vi "ADAM_to_Eng_units.vi"(3 "Ch Description":T1={"Ch Name"="", "Type"="", "Function"=enum."Analogue Input", "Ch State"=enum."On", "Calibration type"="", "A"=0.0, "B"=0.0, "C"=0.0, "D"=0.0, "Comments"="", "Address"={"Main"=0, "Ch."=0, "Sub"=0, "Port Name"=""}, "String"="", "Duty"=65535} {"Duty" format="%016b"; "D" format="%#_5g"; "C" format="%#_5g"; "B" format="%#_5g"; "A" format="%#_5g"}, 5 "Raw":dbl format="%.2f") -> (1 "Calibrated units":dbl format="%.2f", 2 "Comments":string)   [LabVIEW 2021]
uses:
  ADAM Client/Sub VIs/ADAM Controls/Ch_description_ADAM.ctl
  ADAM Client/Sub VIs/ADAM Controls/Module_type_ADAM.ctl
  ADAM Client/Sub VIs/ADAM Controls/Function_ADAM.ctl
  ADAM Client/Sub VIs/ADAM Controls/Channel_State.ctl
  ADAM Client/Sub VIs/ADAM Controls/Calib_type_ADAM.ctl
  ADAM Client/Sub VIs/ADAM Controls/Address.ctl
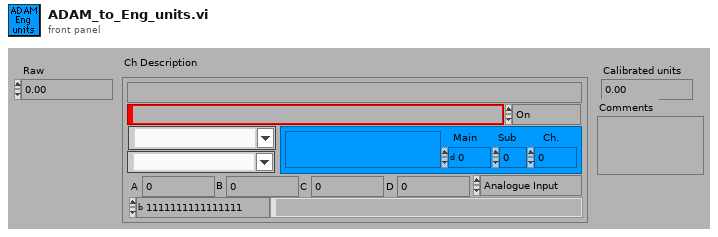
[diagram p1: front panel]
types:
  T1 = typedef "Ch_description_ADAM.ctl" = cluster{"Ch Name":string, "Type":T2, "Function":T3, "Ch State":T4, "Calibration type":T5, "A":dbl, "B":dbl, "C":dbl, "D":dbl, "Comments":string, "Address":T6, "String":string, "Duty":u16}
  T2 = typedef "Module_type_ADAM.ctl" = string
  T3 = typedef "Function_ADAM.ctl" = enum16{"Analogue Input", "Digital Input", "Event counter", "Event rate", "Analogue Output", "Digital Output", "Relay Output"}
  T4 = typedef "Channel_State.ctl" = enum16{"On", "Off", "Always On", "Always Off"}
  T5 = typedef "Calib_type_ADAM.ctl" = string
  T6 = typedef "Address.ctl" = cluster{"Main":i32, "Ch.":i32, "Sub":i32, "Port Name":string}
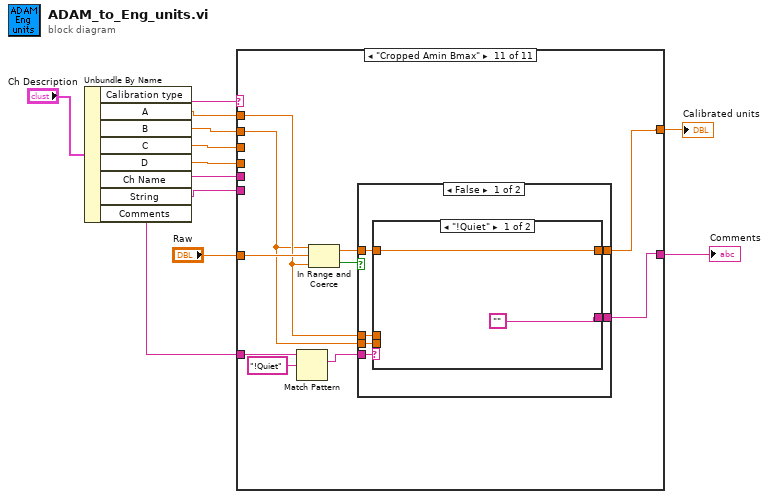
[diagram p0: block diagram]
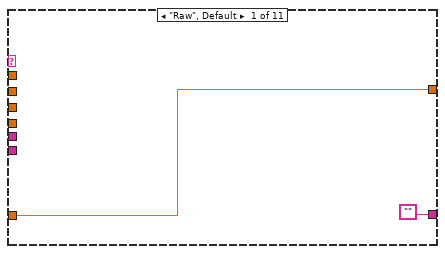
[diagram p2: hidden frame]
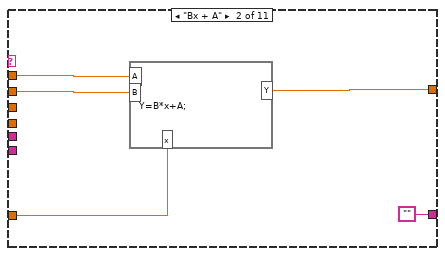
[diagram p3: hidden frame]
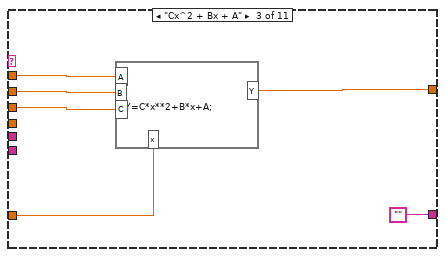
[diagram p4: hidden frame]
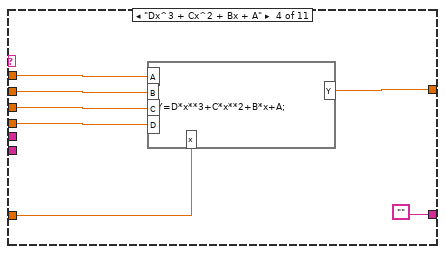
[diagram p5: hidden frame]
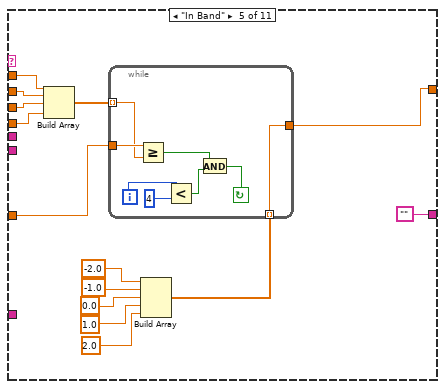
[diagram p6: hidden frame]
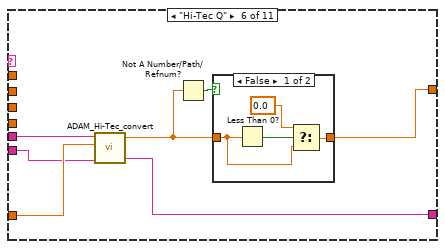
[diagram p7: hidden frame]
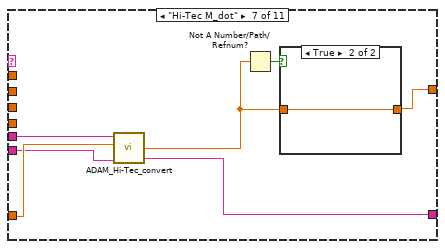
[diagram p9: hidden frame]
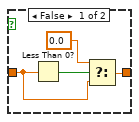
[diagram p10: hidden frame]
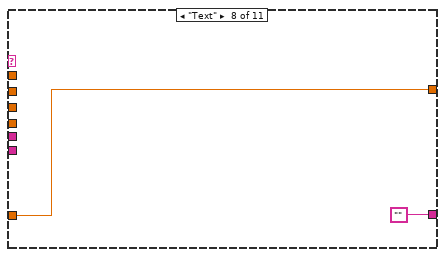
[diagram p11: hidden frame]
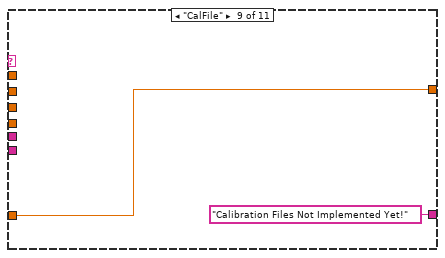
[diagram p12: hidden frame]
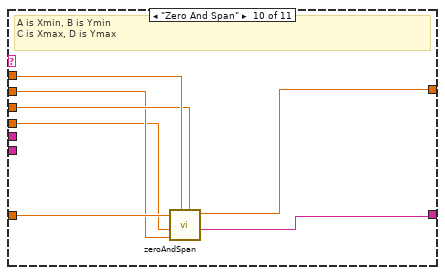
[diagram p13: hidden frame]
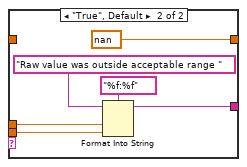
[diagram p14: hidden frame]
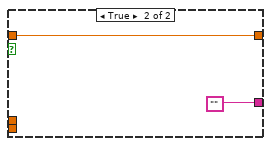
[diagram p15: hidden frame]
diagram:
  n1 = Unbundle By Name("Ch Description") -> ("Calibration type"=w11:T5, "A"=w8:dbl, "B"=w7:dbl, "C"=w6:dbl, "D"=w5:dbl, "Ch Name"=w4:string, "String"=w2:string, "Comments"=w1:string)
  n2 = case shown="\"Cropped Amin Bmax\"" w11 {
    tunnel: [w14 w19 w25 w32 w35 w58 w70 w80 w82 w87 w97] -> w10
    tunnel: "Raw" -> [w14 w16 w21 w27 w42 w60 w72 w80 w82 w89 w99]
    tunnel: w8 -> [_ w18 w24 w31 w46 _ _ _ _ w86 w94]
    tunnel: w7 -> [_ w17 w23 w30 w45 _ _ _ _ w84 w93]
    tunnel: w6 -> [_ _ w22 w29 w44 _ _ _ _ w85 _]
    tunnel: w5 -> [_ _ _ w28 w43 _ _ _ _ w83 _]
    tunnel: w4 -> [_ _ _ _ _ w61 w73 _ _ _ _]
    tunnel: ["" "" "" "" "" w56 w68 "" "Calibration Files Not Implemented Yet!" ("Comments") w88 w95] -> w3
    tunnel: w2 -> [_ _ _ _ _ w55 w67 _ _ _ _]
    tunnel: w1 -> [_ _ _ _ _ _ _ _ _ _ w91]
    frame "Raw", Default {
    }
    frame "Bx + A" {
      n3 = formula code="Y=B*x+A;"("A"=w18, "B"=w17, "x"=w16) -> ("Y"=w19:dbl)
    }
    frame "Cx^2 + Bx + A" {
      n4 = formula code="Y=C*x**2+B*x+A;"("A"=w24, "B"=w23, "C"=w22, "x"=w21) -> ("Y"=w25:dbl)
    }
    frame "Dx^3 + Cx^2 + Bx + A" {
      n5 = formula code="Y=D*x**3+C*x**2+B*x+A;"("A"=w31, "B"=w30, "C"=w29, "D"=w28, "x"=w27) -> ("Y"=w32:dbl)
    }
    frame "In Band" {
      n6 = Build Array(w46, w45, w44, w43) -> (w41:dbl[])
      n7 = Build Array(-2.0, -1.0, 0.0, 1.0, 2.0) -> (w34:dbl[])
      n8 = while {
        tunnel: w34 -> [w52] mode=indexing
        tunnel: [w52] -> w35
        tunnel: w41 -> [w53] mode=indexing
        tunnel: w42 -> [w54]
        i -> [w51]
        stop <- w47 continue-if-true
        n9 = Greater Or Equal?(x=w54, y=w53) -> (x >= y?=w48:bool)
        n10 = Less?(x=w51, y=4) -> (x < y?=w49:bool)
        n11 = And(x=w48, y=w49) -> (x .and. y?=w47:bool)
      }
    }
    frame "Hi-Tec Q" {
      n12 = call "ADAM_Hi-Tec_convert.vi"("Ch Name"=w61, "Raw"=w60, "Channel Read"=w55) -> ("Q release (l/min)"=w57:dbl, "Comments"=w56:string)  [unwired: 1 in, 2 out]
      n13 = Not A Number/Path/Refnum?(number/path/refnum=w57) -> (NaN/Path/Refnum?=w59:bool)
      n14 = case shown="False" w59 {
        tunnel: [w63 w66] -> w58
        tunnel: w57 -> [w64 w66]
        frame False {
          n15 = Less Than 0?(x=w64) -> (x < 0?=w65:bool)
          n16 = Select(t=0.0, s=w65, f=w64) -> (s? t:f=w63:dbl)
        }
        frame True {
        }
      }
    }
    frame "Hi-Tec M_dot" {
      n17 = call "ADAM_Hi-Tec_convert.vi"("Ch Name"=w73, "Raw"=w72, "Channel Read"=w67) -> ("M_dot (kg/min)"=w69:dbl, "Comments"=w68:string)  [unwired: 1 in, 2 out]
      n18 = Not A Number/Path/Refnum?(number/path/refnum=w69) -> (NaN/Path/Refnum?=w71:bool)
      n19 = case shown="True" w71 {
        tunnel: [w75 w78] -> w70
        tunnel: w69 -> [w76 w78]
        frame False {
          n20 = Less Than 0?(x=w76) -> (x < 0?=w77:bool)
          n21 = Select(t=0.0, s=w77, f=w76) -> (s? t:f=w75:dbl)
        }
        frame True {
        }
      }
    }
    frame "Text" {
    }
    frame "CalFile" {
    }
    frame "Zero And Span" {
      # "A is Xmin, B is Ymin\nC is Xmax, D is Ymax"
      n22 = call "zeroAndSpan.vi"("Xmax (100)"=w85, "Xmin (0)"=w86, "Ymin"=w84, "Ymax"=w83, "MeasuredX"=w89) -> ("Message"=w88:string, "calibratedY"=w87:dbl)  [unwired: 4 in, 1 out]
    }
    frame "Cropped Amin Bmax" {
      n23 = Match Pattern(string=w91, regular expression="!Quiet") -> (match substring=w92:string)  [unwired: 1 in, 3 out]
      n24 = In Range and Coerce(upper limit=w93, x=w99, lower limit=w94) -> (coerced(x)=w96:dbl, In Range?=w98:bool)
      n25 = case shown="False" w98 {
        tunnel: [w105 w115] -> w97
        tunnel: w96 -> [w100 w115]
        tunnel: w94 -> [w104 _]
        tunnel: w93 -> [w103 _]
        tunnel: [w102 ""] -> w95
        tunnel: w92 -> [w101 _]
        frame False {
          n26 = case shown="\"!Quiet\"" w101 {
            tunnel: [w107 nan] -> w105
            tunnel: w104 -> [_ w111]
            tunnel: w103 -> [_ w110]
            tunnel: ["" w108] -> w102
            tunnel: w100 -> [w107 _]
            frame "!Quiet" {
            }
            frame "True", Default {
              n27 = Format Into String(format string="%f:%f", initial string="Raw value was outside acceptable range ", w111, w110) -> (resulting string=w108:string)  [unwired: 1 in, 1 out]
            }
          }
        }
        frame True {
        }
      }
    }
  }
  "Calibrated units" <- w10
  "Comments" <- w3
